vi "Get PublicEvents.vi"(8 "error in (no error)":errorcluster, 11 "Application in":refnum<class "Application.lvclass">) -> (0 "error out":errorcluster, 2 "Public Events":T1, 3 "Application out":refnum<class "Application.lvclass">)   [LabVIEW 2019, in "Application.lvclass"]
doc: "Developed by Kevin Thompson\nkevin@thompsonengineering.net\n\nCopyright 2018\nThompson Engineering, LLC"
uses:
  Application.lvclass
  Common/DataTypes/TD Async CmdMsg EventData--cluster.ctl
  DataTypes/Public Events--cluster.ctl
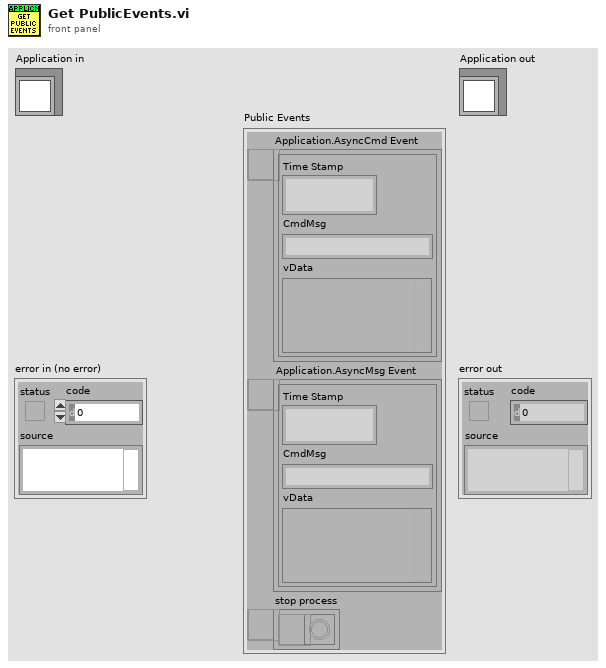
[diagram p1: front panel]
types:
  T1 = typedef "Application.lvclass/Public Events--cluster.ctl" = cluster{"Application.AsyncCmd Event":refnum<user-event>, "Application.AsyncMsg Event":refnum<user-event>, "stop process":refnum<user-event>}
  T2 = typedef "Application.lvclass/ObjData--cluster.ctl" = cluster{"Settings":T3, "Public Events":T1, "Dependency":T4, "ReadData-placeholder":T5, "VISA-placeholder":refnum<visa-resource-name>, "Subsys ClassRefs Dict":T6, "InverterWaveformsQ":T7, "RawDaqDataQ":T8}
  T3 = typedef "Application.lvclass/Settings--cluster.ctl" = cluster{"Simulation":bool}
  T4 = typedef "Application.lvclass/Dependency--cluster.ctl" = cluster{"Config":refnum<class "Config.lvclass">, "Main":refnum<class "Main.lvclass">, "ErrorHandler":refnum<class "ErrorHandler.lvclass">, "DAQ_Engine":refnum<class "DAQ_Engine.lvclass">, "Log_Engine":refnum<class "Log_Engine.lvclass">}
  T5 = typedef "Application.lvclass/Read Data--cluster.ctl" = cluster{"Data":dbl}
  T6 = typedef "TD Dynamic CVT DVR--ref.ctl" = refnum<data-value>
  T7 = typedef "InverterWaveforms--QRef.ctl" = refnum<queue>
  T8 = typedef "RawDAQDataQRef--cluster.ctl" = refnum<queue>
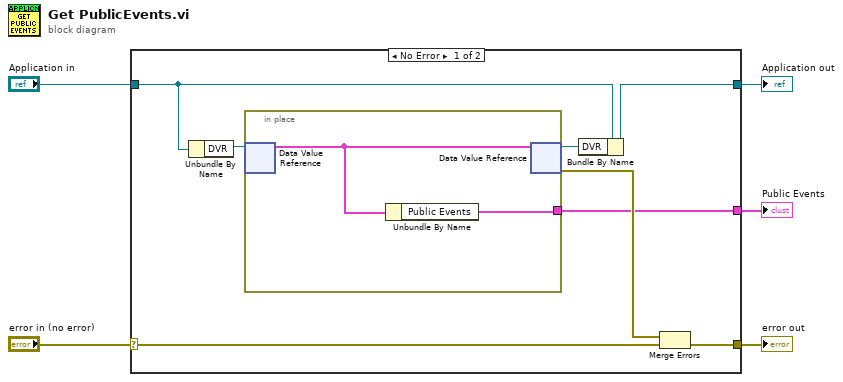
[diagram p0: block diagram]
diagram:
  n1 = case shown="No Error" "error in (no error)" {
    selector: "error in (no error)" -> [w6 w16]
    tunnel: [w7 w16] -> w4
    tunnel: [w10 w17] -> w2
    tunnel: "Application in" -> [w9 w17]
    tunnel: [w8 _] -> w1
    frame No Error {
      n2 = Unbundle By Name(w9) -> ("DVR"=w12:refnum<data-value>)
      n3 = in-place {
        in-place-border: [w14] -> w8
        n4 = in-place-dvr #1(w12) -> (w15:T2)  [unwired: 1 out]
        n5 = Unbundle By Name(w15) -> ("Public Events"=w14:T1)
        n6 = in-place-dvr #1(w15) -> (w13:refnum<data-value>, w11:errorcluster)
      }
      n7 = Bundle By Name(cluster=w9, "DVR"=w13) -> (w10:refnum<class "Application.lvclass">)
      n8 = Merge Errors(w11, w6) -> (w7:errorcluster)
    }
    frame Error {
    }
  }
  "error out" <- w4
  "Application out" <- w2
  "Public Events" <- w1
